vi "PNSGrenzwerteGleich.vi"() -> (3 "ungleich":bool)   [LabVIEW 2020, in "Stoerungen.lvlib"]
uses:
  Stoerungen.lvlib
  PNS/Aktionen FGV Grenzwerte.ctl
  PNS/PNS.lvlib
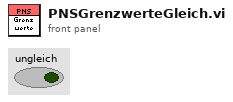
[diagram p1: front panel]
types:
  T1 = typedef "PNS.lvlib/Aktionen FGV Grenzwerte.ctl" = enum16{"lesen", "Grenzw. schreiben", "Anweisungscode", "IP-Adresse"}
  T2 = typedef "Steuerung PNS.lvclass/Anlegengrenzwerte PNS.ctl" = cluster{"Filter:":T3, "Ventilplatte:":T3, "Heizleitung 1:":T3, "Heizleitung 2:":T3, "Heizleitung 3:":T3, "Heizleitung 4:":T3, "Heizleitung 5:":T3, "Heizleitung 6:":T3}
  T3 = typedef "Steuerung PNS.lvclass/Anlagengrenzwerte Parameteranzeige.ctl" = cluster{"Sollwert":T4, "Warn-Min":T4, "Warn-Max":T4, "Abschalt-Min":T4, "Abschalt-Max":T4, "Regler":u16, "AnlagenParameter":string}
  T4 = typedef "Zahlen-Eingabefeld.ctl" = sgl
  T5 = cluster{"Sollwert":T4, "Abschalt-Min":T4, "Abschalt-Max":T4, "Regler":u16}
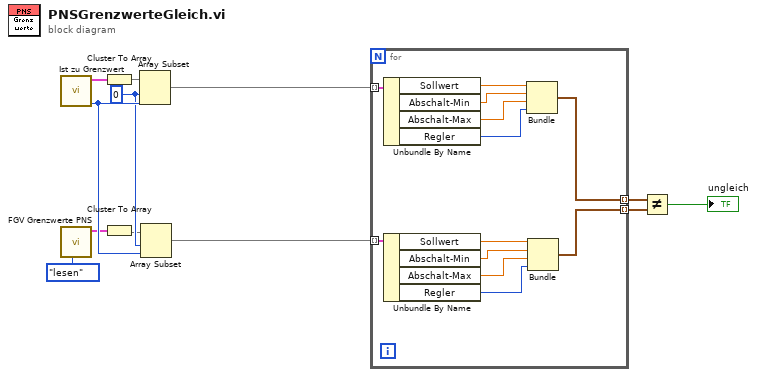
[diagram p0: block diagram]
diagram:
  w11 = 0 ("Index")
  n1 = call "Ist zu Grenzwert.vi"() -> ("maxLoop"=w12:i32, "Grenzwerte Ist"=w7:T2)  [unwired: 10 in]
  n2 = call "FGV Grenzwerte PNS.vi"("Aktionen FGV Grenzwerte"=Aktionen_FGV_Grenzwerte."lesen" ("Aktionen")) -> ("Grenzwerte PNS 2"=w8:T2)  [unwired: 8 in, 2 out]
  n3 = Cluster To Array(cluster=w7) -> (array=w9:T3[])
  n4 = Cluster To Array(cluster=w8) -> (array=w10:T3[])
  n5 = Array Subset(array=w9, index=w11, length=w12) -> (w4:T3[])
  n6 = Array Subset(array=w10, index=w11, length=w12) -> (w5:T3[])
  n7 = for {
    tunnel: w5 -> [w23] mode=indexing
    tunnel: w4 -> [w24] mode=indexing
    tunnel: [w14] -> w3 mode=indexing
    tunnel: [w13] -> w2 mode=indexing
    n8 = Unbundle By Name(w24) -> ("Sollwert"=w22:T4, "Abschalt-Min"=w21:T4, "Abschalt-Max"=w20:T4, "Regler"=w19:u16)
    n9 = Unbundle By Name(w23) -> ("Sollwert"=w18:T4, "Abschalt-Min"=w17:T4, "Abschalt-Max"=w16:T4, "Regler"=w15:u16)
    n10 = Bundle("Sollwert"=w22, "Abschalt-Min"=w21, "Abschalt-Max"=w20, "Regler"=w19) -> (w14:T5)  [unwired: 1 in]
    n11 = Bundle("Sollwert"=w18, "Abschalt-Min"=w17, "Abschalt-Max"=w16, "Regler"=w15) -> (w13:T5)  [unwired: 1 in]
  }
  n12 = Not Equal?(x=w3, y=w2) -> (x != y?=→"ungleich":bool)
